vi "Bundle Script_Properties Remove Unwired.vi"(8 "error in":errorcluster, 11 "Affected Items 2":T1) -> (0 "error out":errorcluster, 2 "Objects":refnum<vi>[](array[refnum]))   [LabVIEW 2023]
uses:
  top/BundleMagic.ctl
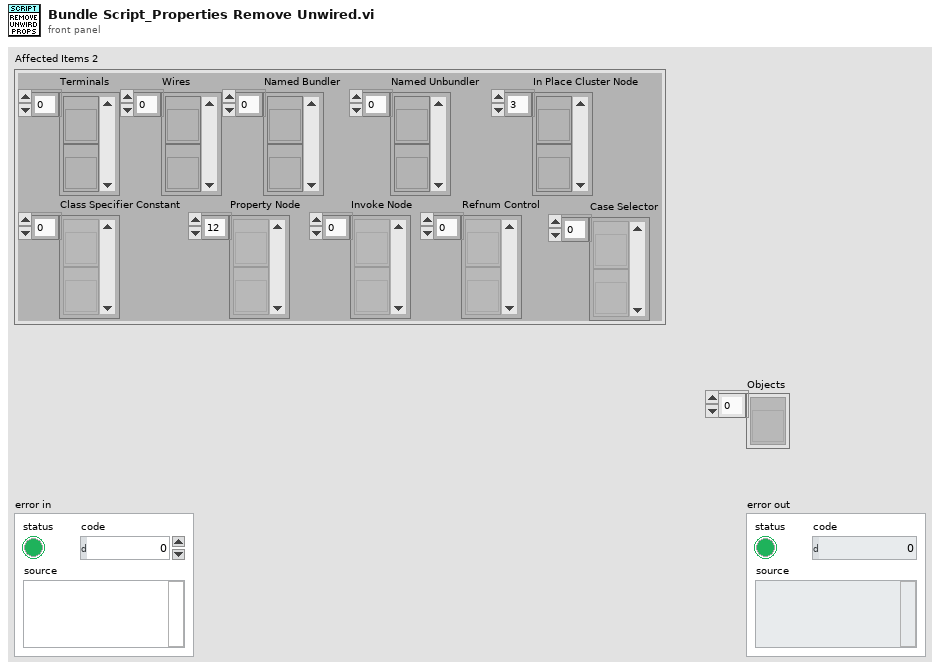
[diagram p1: front panel]
types:
  T1 = typedef "BundleMagic.ctl" = cluster{"Terminals":refnum<vi>[], "Wires":refnum<vi>[], "Named Bundler":refnum<vi>[], "Named Unbundler":refnum<vi>[], "In Place Cluster Node":refnum<vi>[], "Class Specifier Constant":refnum<vi>[], "Property Node":refnum<vi>[], "Invoke Node":refnum<vi>[], "Refnum Control":refnum<vi>[], "Case Selector":refnum<vi>[]}
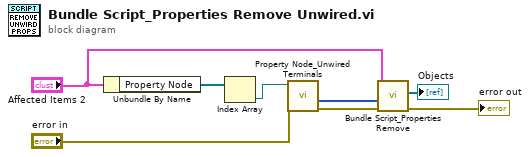
[diagram p0: block diagram]
diagram:
  n1 = Unbundle By Name("Affected Items 2") -> ("Property Node"=w8:refnum<vi>[])
  n2 = Index Array(array=w8) -> (element=w7:refnum<vi>)  [unwired: 1 in]
  n3 = call "Property Node_Unwired Terminals.vi"("error in"="error in", "Property Node Ref"=w7) -> ("error out"=w4:errorcluster, "Unwired Indices For Removal"=w6:i32[])  [unwired: 6 in, 2 out]
  n4 = call "Bundle Script_Properties Remove.vi"("error in"=w4, "Remove Indices"=w6, "Affected Items"="Affected Items 2") -> ("error out"=→"error out":errorcluster, "Objects"=→"Objects":refnum<vi>[])  [unwired: 7 in]
